vi "Assert Check Attendance Table If Exit.vi"() -> ()   [LabVIEW 2015, in "CalAttendance.lvclass"]
uses:
  CalAttendance/CalAttendance.lvclass
  ExcelReader.lvclass
panel:
  out "Fit(False)":bool
  in  "SheetName(\"\")":string="测试"
  in  "Path":path
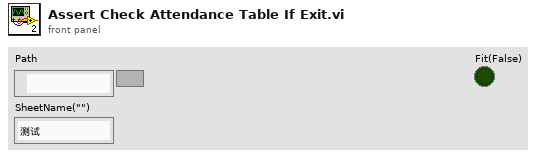
[diagram p1: front panel]
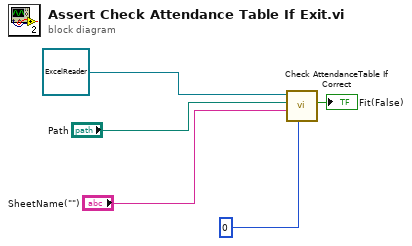
[diagram p0: block diagram]
diagram:
  n1 = call "Check AttendanceTable If Correct.vi"("CurWeek(0)"=0, "SheetName(\"\")"="SheetName(\"\")", "Path"="Path", "ExcelReader in"=refnum<class "ExcelReader.lvclass"> refnum) -> ("Fit(False)"=→"Fit(False)":bool)  [unwired: 5 in, 2 out]
